vi "Load User Plugin.vi"(8 "error in (no error)":errorcluster, 10 "Name or relative path":string, 11 "DSI Reference":refnum<class "DCM-DSI.lvclass">) -> (0 "error out":errorcluster, 2 "Plugin Reference":refnum<class "DCM-DSI.lvclass">, 3 "DSI Reference":refnum<class "DCM-DSI.lvclass">)   [LabVIEW 2016, in "DCM-DSI.lvclass"]
uses:
  DCM-DSI.lvclass
  DCM-DSI.lvclass/DCM-DSI.ctl
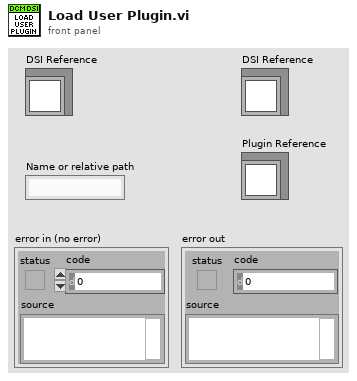
[diagram p1: front panel]
types:
  T1 = cluster{"DCM Ref":refnum<class "DCM - RT.lvclass">, "ExpansionRIO Ref":refnum<data-value>, "DiffIO Results":refnum<data-value>, "DiffIO State":refnum<data-value>, "DiffIO Setup":refnum<data-value>, "EPTx Data":refnum<data-value>, "ESTTL Setup":refnum<data-value>, "Knock Results":refnum<data-value>, "HH Config":refnum<data-value>, "HH Command":refnum<data-value>, "HH Scope Data":refnum<data-value>, "HH Scope Ctr":refnum<data-value>, "HH Status":refnum<data-value>, "DI-A Command":refnum<data-value>, "DI-B Command":refnum<data-value>, "DI-A Profiles":refnum<data-value>, "DI-B Profiles":refnum<data-value>, "DI Scope Data":refnum<data-value>, "DI Scope dt [s]":refnum<data-value>, "DI Scope Ctr":refnum<data-value>, "Pump-A Command":refnum<data-value>, "Pump-B Command":refnum<data-value>, "Skip Fire Setup":refnum<data-value>, "System State":refnum<data-value>}
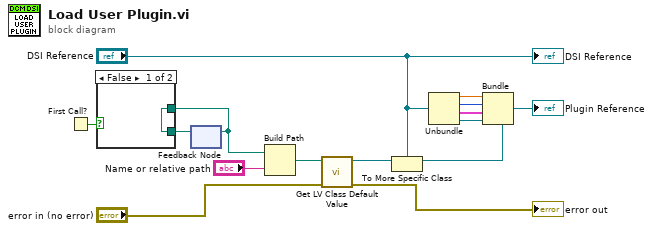
[diagram p0: block diagram]
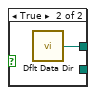
[diagram p2: hidden frame]
diagram:
  n1 = First Call?() -> (First Call?: T/F=w15:bool)
  n2 = feedback #1() -> (w14:path)  [unwired: 1 in]
  n3 = case shown="False" w15 {
    tunnel: [w16 w17] -> w13
    tunnel: w14 -> [w16 _]
    frame False {
    }
    frame True {
      n4 = call <vilib>:"Dflt Data Dir.vi"() -> ("App:Default Data Directory"=w17:path)
    }
  }
  n5 = feedback-in #1(w13) -> ()
  n6 = Build Path(base path=w13, name or relative path="Name or relative path") -> (appended path=w11:path)
  n7 = call <vilib>:"Get LV Class Default Value.vi"("error in (no error)"="error in (no error)", "class path"=w11) -> ("error out"=→"error out":errorcluster, "object"=w9:refnum<class>)  [unwired: 8 in]
  n8 = To More Specific Class(target class="DSI Reference", reference=w9) -> (specific class reference=w6:refnum<class "DCM-DSI.lvclass">)  [unwired: 1 in, 1 out]
  n9 = Unbundle("DSI Reference") -> (w5:dbl, w4:i32, w3:T1, w2:refnum<data-value>)
  n10 = Bundle(cluster=w6, w5, w4, w3, w2) -> (→"Plugin Reference":refnum<class "DCM-DSI.lvclass">)
  "DSI Reference" <- "DSI Reference"
